vi "CameraConnectCheck.vi"(2 "错误输入（无错误）":errorcluster, 3 "是否通信检查":bool) -> (0 "通信正常？":bool, 1 "error out":errorcluster)   [LabVIEW 2018]
uses:
  VsyCam.dll
panel:
  out "采集套接":i32
  out "控制套接":i32
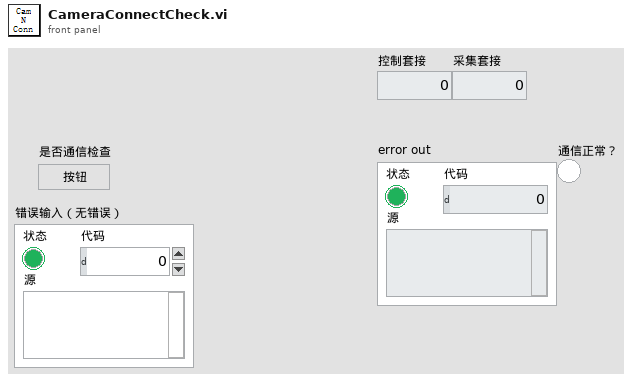
[diagram p1: front panel]
types:
  T1 = typedef "IMAQ Image.ctl" = refnum<image>
  T2 = cluster{"示波器":cluster{"Channel (0:Channel 1)":enum16{"Channel 1", "Channel 2", "Channel 3", "Channel 4"}, "电压范围":dbl, "触发电压":dbl, "时间范围":dbl, " 示波器VISA":refnum<visa-resource-name>, "时间范围 标签":u64, "电压范围 标签":u64, "触发电压 标签":u64}, "光谱仪":cluster{"Channel (0:Channel 1)":enum16{"Channel 1", "Channel 2", "Channel 3", "Channel 4"}, "电压范围":u64, "触发电压":u64, "时间范围":u64}, " 近场相机":cluster{"曝光时间":dbl, "模拟增益":i32, "控制套接字":i32, "IP 地址":string, " 采集套接字":i32, "  版本号":i32, "ImageData":T1, "  增益最大":i32, "  增益最小":i32, " 曝光最大":i32, " 曝光最小":i32, " 帧速":i32, " 同步切换":i32, "  曝光缩放":i32}, " 偏振仪":cluster{"电压范围":u64, "触发电压":u64, "时间范围":u64, "波长范围":enum16{"可见光 400-700nm", "近红外 700-1100nm"}, "可见光偏振测量仪VISA":refnum<visa-resource-name>, "近红外偏振测量仪VISA":refnum<visa-resource-name>}, " 功率计":cluster{"通道":enum16{"Channel 1", "Channel 2"}, "工作波长":u32, "单位":u64, "时间范围":u64, "IP地址":string, "端口":u32}, "能量计":cluster{"通道":enum16{"Channel 1", "Channel 2"}, "工作波长":u32, "单位":u64, "时间范围":u64, "IP地址":string, "端口":u32, "能量计量程":enum16{"200uJ", "20uJ", "2uJ", "200nJ"}}, "电机":cluster{"Channel (0:Channel 1)":enum16{"Channel 1", "Channel 2", "Channel 3", "Channel 4"}, "电压范围":u64, "触发电压":u64, "时间范围":u64}, " 远场相机":cluster{"曝光时间":i32, "模拟增益":i32, "控制套接字":i32, "IP 地址":string, " 采集套接字":i32, "  版本号":i32, "ImageData":T1, "  增益最大":i32, "  增益最小":i32, " 曝光最大":i32, " 曝光最小":i32, " 帧速":i32, " 同步切换":i32, "  曝光缩放":i32}}
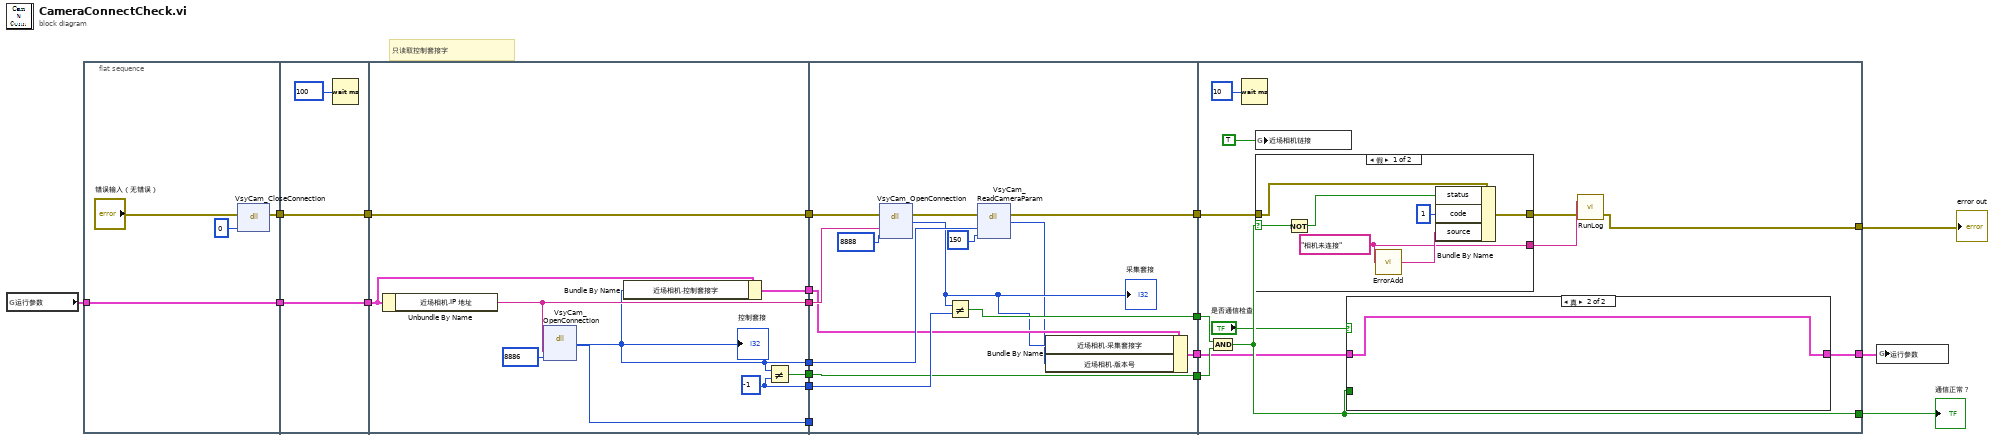
[diagram p0: block diagram]
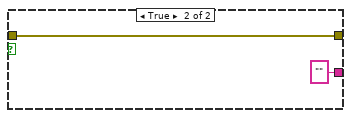
[diagram p2: hidden frame]
diagram:
  # "只读取控制套接字"
  n1 = global read "参数.vi" "运行参数"() -> (w4:T2)
  n2 = flat-sequence {
    tunnel: w4 -> [w23]
    tunnel: [w23] -> w19
    tunnel: [w21] -> w5
    tunnel: w19 -> [w25]
    tunnel: [w25] -> w18
    tunnel: [w24] -> w6
    tunnel: w5 -> [w24]
    tunnel: [w33] -> w17
    tunnel: [w32] -> w16
    tunnel: [w28] -> w15
    tunnel: [w28] -> w14
    tunnel: w18 -> [w27]
    tunnel: [w31] -> w13
    tunnel: [w30] -> w12
    tunnel: [w29] -> w7
    tunnel: w6 -> [w29]
    tunnel: w17 -> [w47]
    tunnel: [w46] -> w11
    tunnel: w16 -> [w46]
    tunnel: [w45] -> w10
    tunnel: w15 -> [_]
    tunnel: w14 -> [w44]
    tunnel: w13 -> [w42]
    tunnel: w12 -> [w41]
    tunnel: [w38] -> w9
    tunnel: [w35] -> w8
    tunnel: w7 -> [w37]
    tunnel: w11 -> [w60]
    tunnel: w10 -> [w59]
    tunnel: w9 -> [w53]
    tunnel: w8 -> [w57]
    tunnel: [w56] -> w3
    tunnel: [w52] -> w2
    tunnel: [w49] -> w1
    frame #0 {
      n3 = dll-call lib="PTH2?abs D做的项目航天测量软件相机\nVsyCam.dll" fn="VsyCam_CloseConnection"(error in="错误输入（无错误）", "sockFd"=0) -> (error out=w21:errorcluster)  [unwired: 4 in, 1 out]
    }
    frame #1 {
      n4 = Wait (ms)(milliseconds to wait=u32 100 ("等待时间（毫秒）")) -> ()  [unwired: 1 out]
    }
    frame #2 {
      w33 = -1
      n5 = Unbundle By Name(w27) -> ("近场相机.IP 地址"=w31:string)
      n6 = dll-call lib="PTH2?abs D做的项目航天测量软件相机\nVsyCam.dll" fn="VsyCam_OpenConnection"("ip"=w31, "port"=8886) -> ("返回类型"=w28:i32)  [unwired: 5 in, 2 out]
      "控制套接" <- w28
      n7 = Bundle By Name(cluster=w27, "近场相机.控制套接字"=w28) -> (w30:T2)
      n8 = Not Equal?(x=w28, y=w33) -> (x != y?=w32:bool)
    }
    frame #3 {
      n9 = dll-call lib="PTH2?abs D做的项目航天测量软件相机\nVsyCam.dll" fn="VsyCam_OpenConnection"(error in=w37, "ip"=w42, "port"=8888) -> (error out=w36:errorcluster, "返回类型"=w40:i32)  [unwired: 4 in, 1 out]
      "采集套接" <- w40
      n10 = Not Equal?(x=w40, y=w47) -> (x != y?=w45:bool)
      n11 = dll-call lib="PTH2?abs D做的项目航天测量软件相机\nVsyCam.dll" fn="VsyCam_ReadCameraParam"(error in=w36, "sockFd"=w44, "cmd"=150) -> (error out=w35:errorcluster, "返回类型"=w39:i32)  [unwired: 4 in, 1 out]
      n12 = Bundle By Name(cluster=w41, "近场相机.采集套接字"=w40, "近场相机.版本号"=w39) -> (w38:T2)
    }
    frame #4 {
      n13 = And(x=w59, y=w60) -> (x .and. y?=w56:bool)
      n14 = Wait (ms)(milliseconds to wait=u32 10 ("等待时间（毫秒）")) -> ()  [unwired: 1 out]
      n15 = global write "globalMessage.vi" "近场相机链接"(TRUE) -> ()
      n16 = case shown="假" w56 {
        selector: w56 -> [w66 _]
        tunnel: w57 -> [w67 w69]
        tunnel: [w62 w69] -> w50
        tunnel: [w61 "" ("source")] -> w51
        frame False {
          w61 = "相机未连接" ("source")
          n17 = Not(x=w66) -> (.not. x?=w65:bool)
          n18 = call "ErrorAdd.vi"("source"=w61) -> ("Errorout Souce"=w63:string)
          n19 = Bundle By Name(cluster=w67, "status"=w65, "code"=1, "source"=w63) -> (w62:errorcluster)
        }
        frame True {
        }
      }
      n20 = case shown="真" "是否通信检查" {
        tunnel: w56 -> [_ _]
        tunnel: w53 -> [w70 w71]
        tunnel: [w70 w71] -> w52
        frame False {
        }
        frame True {
        }
      }
      n21 = call "RunLog.vi"("error in"=w50, "Message"=w51) -> ("error out"=w49:errorcluster)  [unwired: 1 in]
    }
  }
  n22 = global write "参数.vi" "运行参数"(w2) -> ()
  "通信正常？" <- w3
  "error out" <- w1
